vi "GetPlotColors.vi"(8 "ErrorIn(No Error)":errorcluster caption="entrée d'erreur (pas d'erreur)", 9 "Color2In":u32, 10 "Color1In":u32, 11 "ColorIndex":i32) -> (0 "sortie d'erreur":errorcluster, 1 "Color2Out":u32, 2 "Color1Out":u32, 3 "AutoColor":bool)   [LabVIEW 2012]
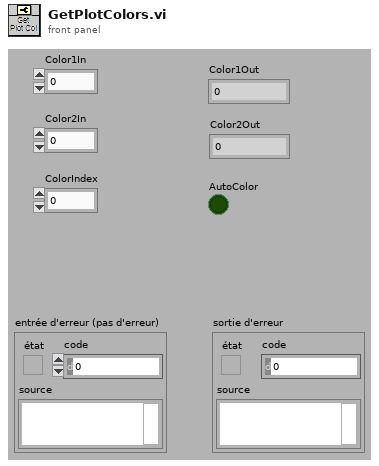
[diagram p1: front panel]
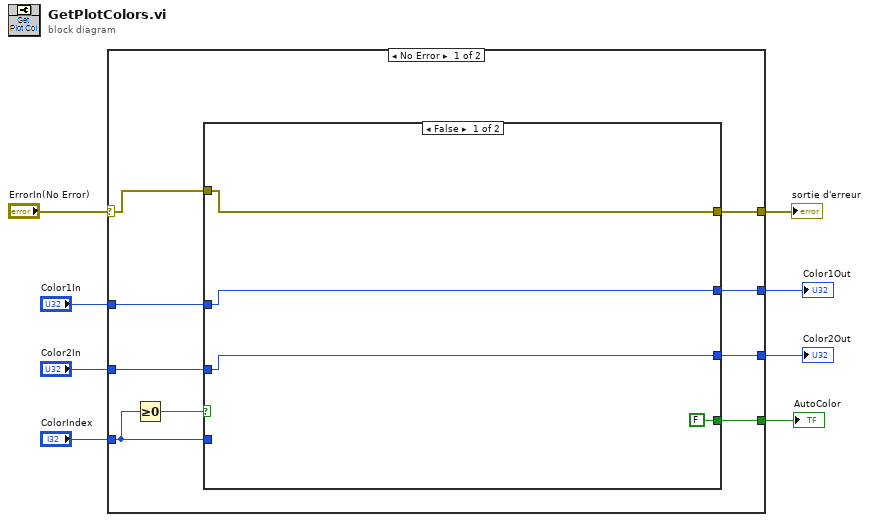
[diagram p0: block diagram]
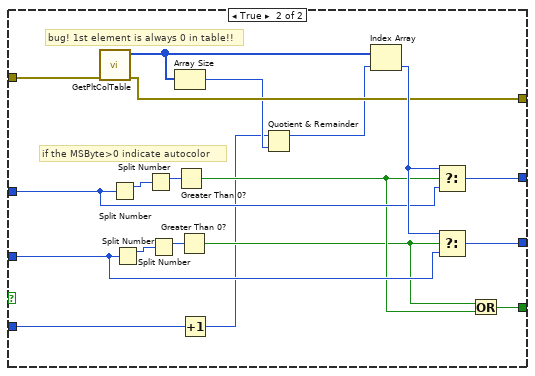
[diagram p2: hidden frame]
diagram:
  n1 = case shown="No Error" "ErrorIn(No Error)" {
    selector: "ErrorIn(No Error)" -> [w12 w41]
    tunnel: [w11 w41] -> w7
    tunnel: "Color1In" -> [w16 _]
    tunnel: "Color2In" -> [w17 _]
    tunnel: "ColorIndex" -> [w10 _]
    tunnel: [w15 _] -> w3
    tunnel: [w14 _] -> w2
    tunnel: [w13 _] -> w1
    frame No Error {
      n2 = Greater Or Equal To 0?(x=w10) -> (x >= 0?=w9:bool)
      n3 = case shown="False" w9 {
        tunnel: w17 -> [w20 w35]
        tunnel: w16 -> [w21 w34]
        tunnel: [w21 w33] -> w15
        tunnel: [w20 w32] -> w14
        tunnel: [FALSE w29] -> w13
        tunnel: w12 -> [w18 w28]
        tunnel: [w18 w27] -> w11
        tunnel: w10 -> [_ w22]
        frame False {
        }
        frame True {
          # "bug! 1st element is always 0 in table!!"
          # "if the MSByte>0 indicate autocolor"
          n4 = call "GetPltColTable.vi"("ErrorIn(No Error)"=w28) -> ("sortie d'erreur"=w27:errorcluster, "Color Table"=w26:u32[])  [unwired: 9 in]
          n5 = Split Number(x=w34) -> (hi(x)=w40:u16)  [unwired: 1 out]
          n6 = Split Number(x=w35) -> (hi(x)=w37:u16)  [unwired: 1 out]
          n7 = Split Number(x=w40) -> (hi(x)=w39:u8)  [unwired: 1 out]
          n8 = Split Number(x=w37) -> (hi(x)=w38:u8)  [unwired: 1 out]
          n9 = Array Size(array=w26) -> (size(s)=w25:i32)
          n10 = Greater Than 0?(x=w39) -> (x > 0?=w31:bool)
          n11 = Greater Than 0?(x=w38) -> (x > 0?=w30:bool)
          n12 = Increment(x=w22) -> (x+1=w24:i32)
          n13 = Quotient & Remainder(x=w24, y=w25) -> (x-y*floor(x/y)=w23:i32)  [unwired: 1 out]
          n14 = Index Array(array=w26, index=w23) -> (element=w36:u32)
          n15 = Select(t=w36, s=w31, f=w34) -> (s? t:f=w33:u32)
          n16 = Select(t=w36, s=w30, f=w35) -> (s? t:f=w32:u32)
          n17 = Or(x=w30, y=w31) -> (x .or. y?=w29:bool)
        }
      }
    }
    frame Error {
    }
  }
  "sortie d'erreur" <- w7
  "Color1Out" <- w3
  "Color2Out" <- w2
  "AutoColor" <- w1
